vi "FGen Simulated_Create.vi"(8 "Error In":errorcluster, 10 "IConfigure.lvclass":refnum<class "IConfigure.lvclass">, 11 "reference in":refnum<class "FGen Simulated.lvclass">) -> (0 "Error Out":errorcluster, 3 "reference out":refnum<class "FGen Simulated.lvclass">)   [LabVIEW 2023, in "FGen Simulated.lvlib" / "FGen Simulated.lvclass"]
uses:
  FGen Simulated.lvclass
  FGen Simulated.lvclass/FGen Simulated.ctl
  FGen Base/FGen Base.lvclass
  D:/git/HAL/HAL GOOP4/FGen/FGen Base/FGen Base.lvclass
  D:/git/HAL/HAL GOOP4/Instrument Base/Instrument Base.lvclass
  D:/git/HAL/HAL GOOP4/FGen/FGen Simulated/FGen Simulated.lvclass
  Interfaces/IConfigure/IConfigure.lvclass
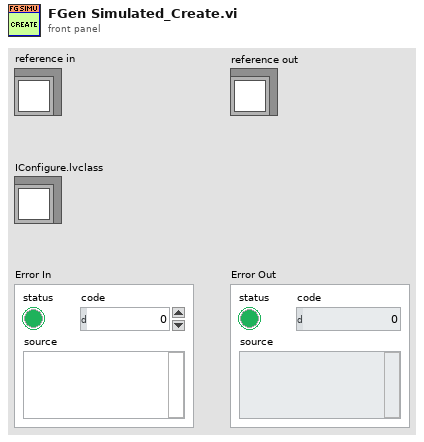
[diagram p1: front panel]
types:
  T1 = typedef "G4SubTemplate_Simple_4x4x4.lvclass/ObjectAttributes.ctl" = cluster{"Attribute1":dbl}
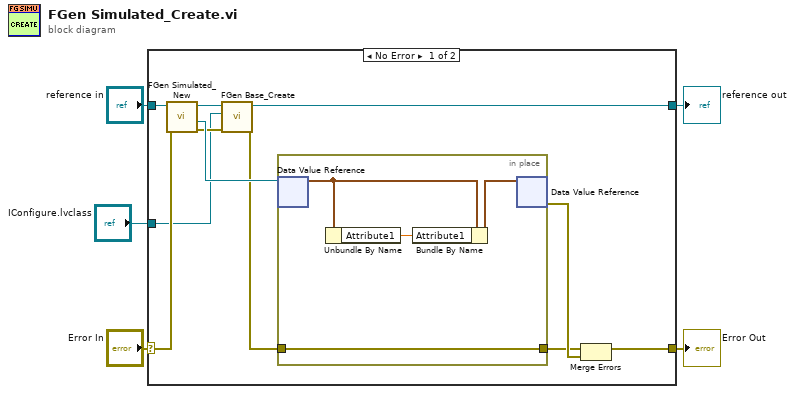
[diagram p0: block diagram]
diagram:
  n1 = case shown="No Error" "Error In" {
    selector: "Error In" -> [w12 w22]
    tunnel: [w10 w22] -> w4
    tunnel: "reference in" -> [w14 w21]
    tunnel: [w9 w21] -> w2
    tunnel: "IConfigure.lvclass" -> [w6 _]
    frame No Error {
      n2 = call "FGen Simulated_New.vi"("Error In"=w12, "reference in"=w14) -> ("Error Out"=w13:errorcluster, "DVRRefOut"=w16:refnum<data-value>, "reference out"=w15:refnum<class "FGen Simulated.lvclass">)  [unwired: 6 in, 1 out]
      n3 = call "FGen Base_Create.vi"("Error In"=w13, "IConfigure.lvclass"=w6, "reference in"=w15) -> ("Error Out"=w8:errorcluster, "reference out"=w9:refnum<class "FGen Simulated.lvclass">)  [unwired: 7 in]
      n4 = in-place {
        in-place-border: w8 -> [w17]
        in-place-border: [w17] -> w7
        n5 = in-place-dvr #1(w16) -> (w19:T1)  [unwired: 1 out]
        n6 = Unbundle By Name(w19) -> ("Attribute1"=w18:dbl)
        n7 = Bundle By Name(cluster=w19, "Attribute1"=w18) -> (w20:T1)
        n8 = in-place-dvr #1(w20) -> (w11:errorcluster)  [unwired: 1 out]
      }
      n9 = Merge Errors(w7, w11) -> (w10:errorcluster)
    }
    frame Error {
    }
  }
  "Error Out" <- w4
  "reference out" <- w2
